vi "Recurse Control References.vi"(8 "error in (no error)":errorcluster, 11 "Ctl Refnum":refnum<vi>) -> (0 "error out":errorcluster, 3 "Control References":T1[](array[typedef]))   [LabVIEW 2023, in "Engine.lvlib" / "Engine.lvclass"]
uses:
  Library/Engine.lvclass
  Custom Controls/Control Reference.ctl
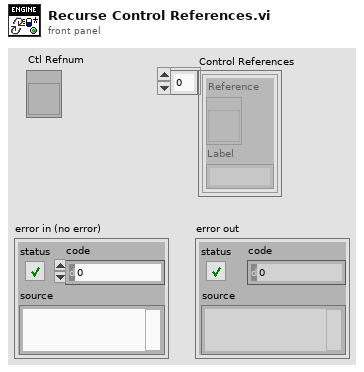
[diagram p1: front panel]
types:
  T1 = typedef "Engine.lvlib/Engine.lvclass/Control Reference.ctl" = cluster{"Reference":refnum<vi>, "Label":string}
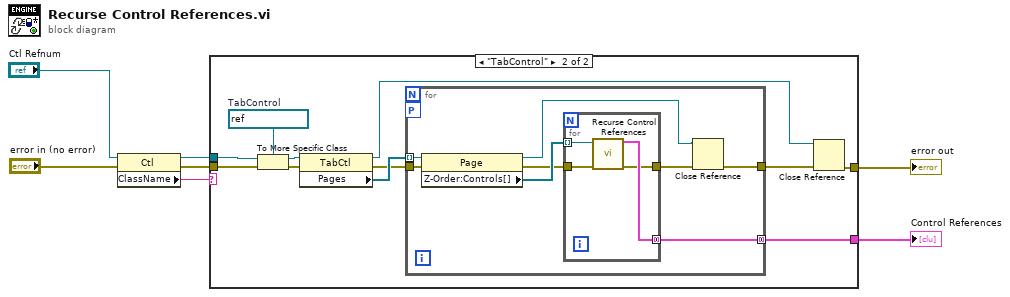
[diagram p0: block diagram]
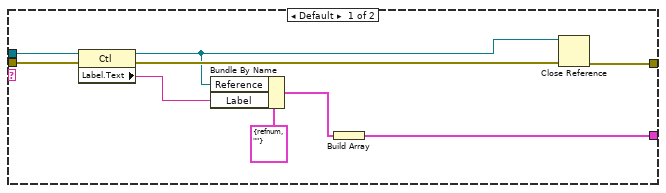
[diagram p2: hidden frame]
diagram:
  n1 = property on="Property Node" class="Ctl"(reference="Ctl Refnum", error in="error in (no error)") -> (reference out=w5:refnum<vi>, error out=w1:errorcluster, "ClassName"=w6:string)
  n2 = case shown="\"TabControl\"" w6 {
    tunnel: w5 -> [w16 w27]
    tunnel: [w15 w22] -> w4
    tunnel: w1 -> [w13 w18]
    tunnel: [w14 w19] -> w3
    frame Default {
      n3 = property on="Property Node" class="Ctl"(reference=w16, error in=w13) -> (reference out=w10:refnum<vi>, error out=w12:errorcluster, "Label.Text"=w11:string)
      n4 = Bundle By Name(cluster=T1 {"Reference"=refnum, "Label"=""} ("Control Def"), "Reference"=w10, "Label"=w11) -> (w9:T1)
      n5 = Build Array(w9) -> (w15:T1[])
      n6 = Close Reference(reference=w10, error in (no error)=w12) -> (error out=w14:errorcluster)
    }
    frame "TabControl" {
      w26 = refnum<vi> refnum  # TabControl
      n7 = To More Specific Class(target class=w26, reference=w27, error in=w18) -> (specific class reference=w25:refnum<vi>, error out=w24:errorcluster)
      n8 = property on="Property Node" class="TabCtl"(reference=w25, error in=w24) -> (reference out=w20:refnum<vi>, error out=w17:errorcluster, "Pages"=w23:refnum<vi>[])
      n9 = for {
        tunnel: w23 -> [w35] mode=indexing
        tunnel: [w33] -> w22 mode=concatenating
        workers-P: _ -> [_]
        tunnel: w17 -> [w29]
        tunnel: [w32] -> w21
        n10 = property on="Property Node" class="Page"(reference=w35, error in=w29) -> (reference out=w30:refnum<vi>, error out=w28:errorcluster, "Z-Order:Controls[]"=w34:refnum<vi>[])
        n11 = for {
          tunnel: w34 -> [w39] mode=indexing
          tunnel: [w38] -> w33 mode=concatenating
          tunnel: w28 -> [w37]
          tunnel: [w36] -> w31
          n12 = call "Recurse Control References.vi"("error in (no error)"=w37, "Ctl Refnum"=w39) -> ("error out"=w36:errorcluster, "Control References"=w38:T1[])  [unwired: 8 in]
        }
        n13 = Close Reference(reference=w30, error in (no error)=w31) -> (error out=w32:errorcluster)
      }
      n14 = Close Reference(reference=w20, error in (no error)=w21) -> (error out=w19:errorcluster)
    }
  }
  "Control References" <- w4
  "error out" <- w3
